vi "Form_recomendation_str.vi"(1 "Recomendation_arr":T1(array[cluster])) -> (0 "Recomendation_str":string)   [LabVIEW 2020]
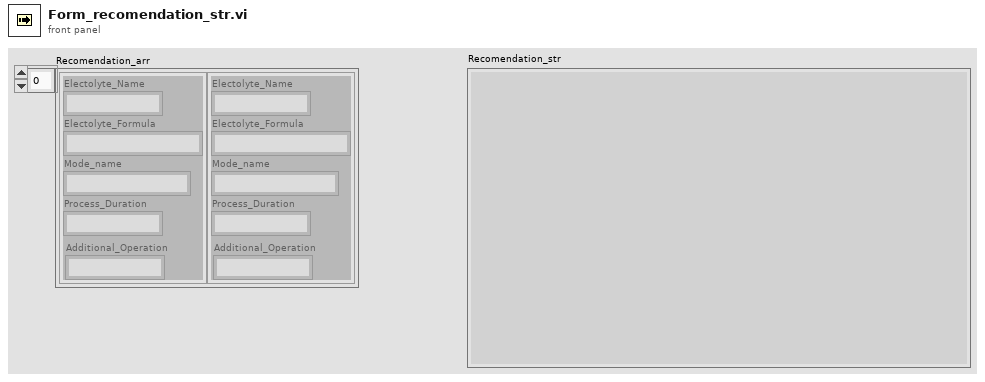
[diagram p1: front panel]
types:
  T1 = cluster{"Electolyte_Name":string, "Electolyte_Formula":string, "Mode_name":string, "Process_Duration":string, "Additional_Operation":string}[]
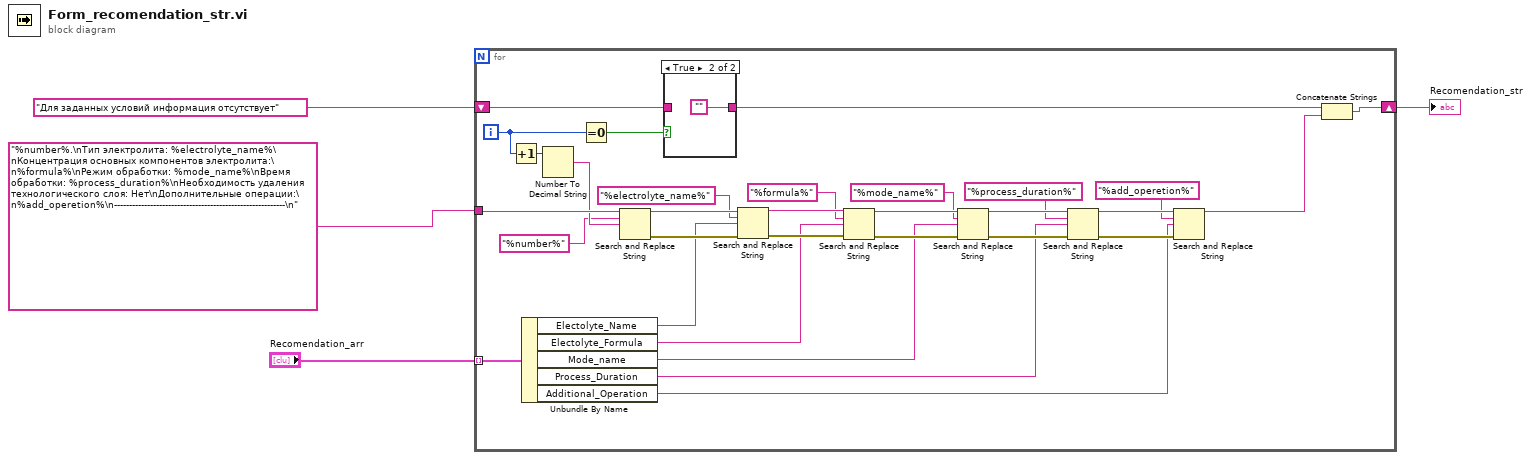
[diagram p0: block diagram]
diagram:
  n1 = for {
    tunnel: "Recomendation_arr" -> [w35] mode=indexing
    tunnel: "%number%.\nТип электролита: %electrolyte_name%\nКонцентрация основных компонентов электролита:\n%formula%\nРежим обработки: %mode_name%\nВремя обработки: %process_duration%\nНеобходимость удаления технологического слоя: Нет\nДополнительные операции:\n%add_operetion%\n---------------------------------------------------------\n" ("Recommendation") -> [w31]
    shift-right: [w32] -> w1
    shift-left: "Для заданных условий информация отсутствует" -> [w34]
    i -> [w5]
    n2 = Increment(x=w5) -> (x+1=w29:i32)
    n3 = Unbundle By Name(w35) -> ("Electolyte_Name"=w24:string, "Electolyte_Formula"=w20:string, "Mode_name"=w16:string, "Process_Duration"=w12:string, "Additional_Operation"=w8:string)
    n4 = Number To Decimal String(number=w29) -> (decimal integer string=w30:string)  [unwired: 1 in]
    n5 = Equal To 0?(x=w5) -> (x = 0?=w6:bool)
    n6 = Search and Replace String(input string=w31, search string="%number%", replace string=w30) -> (result string=w27:string, error out=w26:errorcluster)  [unwired: 5 in, 2 out]
    n7 = case shown="True" w6 {
      tunnel: w34 -> [w36 _]
      tunnel: [w36 ""] -> w33
      frame False {
      }
      frame True {
      }
    }
    n8 = Search and Replace String(input string=w27, search string="%electrolyte_name%", replace string=w24, error in=w26) -> (result string=w23:string, error out=w22:errorcluster)  [unwired: 4 in, 2 out]
    n9 = Search and Replace String(input string=w23, search string="%formula%", replace string=w20, error in=w22) -> (result string=w18:string, error out=w19:errorcluster)  [unwired: 4 in, 2 out]
    n10 = Search and Replace String(input string=w18, search string="%mode_name%", replace string=w16, error in=w19) -> (result string=w14:string, error out=w15:errorcluster)  [unwired: 4 in, 2 out]
    n11 = Search and Replace String(input string=w14, search string="%process_duration%", replace string=w12, error in=w15) -> (result string=w10:string, error out=w11:errorcluster)  [unwired: 4 in, 2 out]
    n12 = Search and Replace String(input string=w10, search string="%add_operetion%", replace string=w8, error in=w11) -> (result string=w7:string)  [unwired: 4 in, 3 out]
    n13 = Concatenate Strings(w33, w7) -> (w32:string)
  }
  "Recomendation_str" <- w1
